vi "DescribeTextField.vi"(0 "XRef":T15, 1 "ID":T3, 2 "State In":T14={"Value"=1415139397}) -> (14 "Text Field Info":T2, 15 "Fatal Error Out":T1)   [LabVIEW 2018, in "Resource Manipulation.lvlib" / "Type ID Constant.xnode"]
uses:
  Type ID Constant.xnode
  <vilib>/XNodeSupport/XNodeXNodeRef.ctl
  <vilib>/XNodeSupport/XNodeString.ctl
  State.ctl
  <vilib>/XNodeSupport/XNodeTextFieldInfo.ctl
  <vilib>/XNodeSupport/XNodeRect32.ctl
  <vilib>/XNodeSupport/XNodeInt.ctl
  <vilib>/XNodeSupport/XNodeJustification.ctl
  <vilib>/XNodeSupport/XNodeHorizontal.ctl
  <vilib>/XNodeSupport/XNodeVertical.ctl
  <vilib>/XNodeSupport/XNodeColor.ctl
  <vilib>/XNodeSupport/XNodeFont.ctl
  <vilib>/XNodeSupport/XNodeUserFont.ctl
  <vilib>/XNodeSupport/XNodeUInt.ctl
  <vilib>/XNodeSupport/XNodeBool.ctl
  <vilib>/XNodeSupport/XNodeErrorCluster.ctl
  <vilib>/XNodeSupport/NI_XNodeSupport.lvlib
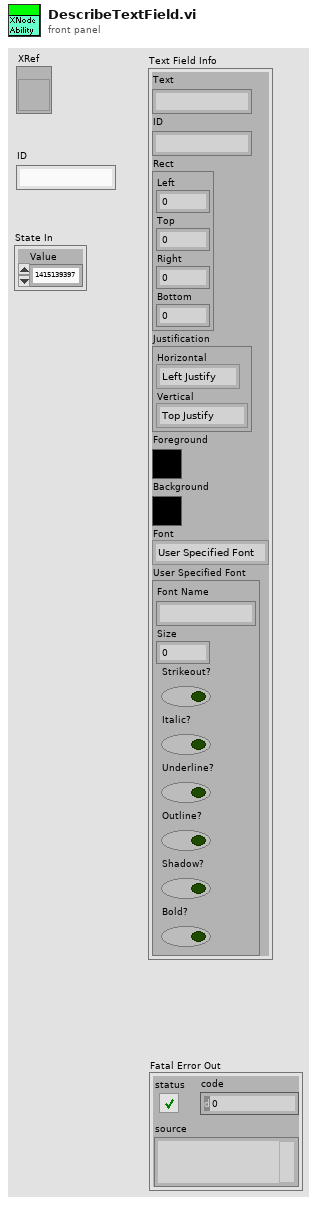
[diagram p1: front panel]
types:
  T1 = typedef "NI_XNodeSupport.lvlib/XNodeErrorCluster.ctl" = errorcluster
  T2 = typedef "NI_XNodeSupport.lvlib/XNodeTextFieldInfo.ctl" = cluster{"Text":T3, "ID":T3, "Rect":T4, "Justification":T6, "Foreground":T9, "Background":T9, "Font":T10, "User Specified Font":T11}
  T3 = typedef "NI_XNodeSupport.lvlib/XNodeString.ctl" = string
  T4 = typedef "NI_XNodeSupport.lvlib/XNodeRect32.ctl" = cluster{"Left":T5, "Top":T5, "Right":T5, "Bottom":T5}
  T5 = typedef "NI_XNodeSupport.lvlib/XNodeInt.ctl" = i32
  T6 = typedef "NI_XNodeSupport.lvlib/XNodeJustification.ctl" = cluster{"Horizontal":T7, "Vertical":T8}
  T7 = typedef "NI_XNodeSupport.lvlib/XNodeHorizontal.ctl" = enum32{"Left Justify", "Right Justify", "CenterJustify"}
  T8 = typedef "NI_XNodeSupport.lvlib/XNodeVertical.ctl" = enum32{"Top Justify", "Bottom Justify", "CenterJustify"}
  T9 = typedef "NI_XNodeSupport.lvlib/XNodeColor.ctl" = u32
  T10 = typedef "NI_XNodeSupport.lvlib/XNodeFont.ctl" = enum32{"User Specified Font", "Application Font", "System Font", "Dialog Font"}
  T11 = typedef "NI_XNodeSupport.lvlib/XNodeUserFont.ctl" = cluster{"Font Name":T3, "Size":T12, "Strikeout?":T13, "Italic?":T13, "Underline?":T13, "Outline?":T13, "Shadow?":T13, "Bold?":T13}
  T12 = typedef "NI_XNodeSupport.lvlib/XNodeUInt.ctl" = u32
  T13 = typedef "NI_XNodeSupport.lvlib/XNodeBool.ctl" = bool
  T14 = typedef "Resource Manipulation.lvlib/Type ID Constant.xnode/State.ctl" = cluster{"Value":u32}
  T15 = typedef "NI_XNodeSupport.lvlib/XNodeXNodeRef.ctl" = refnum<vi>
  T16 = typedef "LVBoundsTypeDef.ctl" = cluster{"Width":u32, "Height":u32}
  T17 = cluster{"left":i16, "top":i16, "right":i16, "bottom":i16}
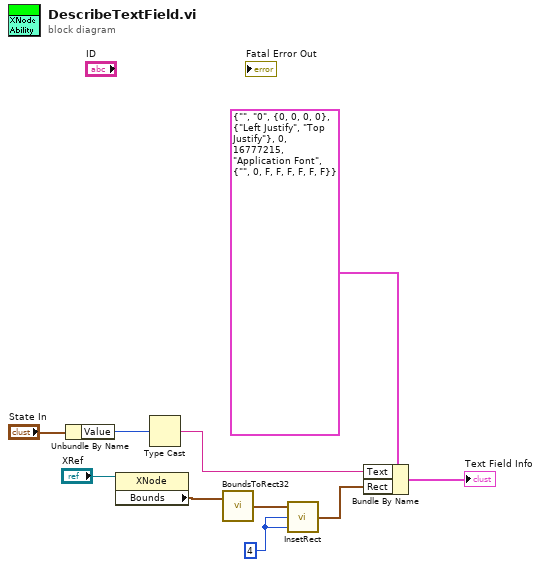
[diagram p0: block diagram]
diagram:
  w7 = i16 4
  n1 = Unbundle By Name("State In") -> ("Value"=w2:u32)
  n2 = property class="XNode"(reference="XRef") -> ("Bounds"=w6:T16)  [unwired: 1 in, 2 out]
  n3 = Type Cast(x=w2) -> (*(type *) &x=w1:string)  [unwired: 1 in]
  n4 = call <vilib>:"BoundsToRect32.vi"("Bounds"=w6) -> ("Rect32"=w5:T4)  [unwired: 1 in]
  n5 = call <vilib>:"InsetRect.vi"("dv"=w7, "dh"=w7, "rect"=w5) -> ("inset rect"=w4:T17)
  n6 = Bundle By Name(cluster=T2 {"Text"="", "ID"="0", "Rect"={"Left"=0, "Top"=0, "Right"=0, "Bottom"=0}, "Justification"={"Horizontal"=enum."Left Justify", "Vertical"=enum."Top Justify"}, "Foreground"=0, "Background"=16777215, "Font"=enum."Application Font", "User Specified Font"={"Font Name"="", "Size"=0, "Strikeout?"=FALSE, "Italic?"=FALSE, "Underline?"=FALSE, "Outline?"=FALSE, "Shadow?"=FALSE, "Bold?"=FALSE}} ("Text Field Info"), "Text"=w1, "Rect"=w4) -> (→"Text Field Info":T2)
